vi "Get Bounds.vi"(8 "error in (no error)":errorcluster, 11 "Shape in":refnum<class "Shape.lvclass">) -> (0 "error out":errorcluster, 2 "Bounds":T1, 3 "Shape out":refnum<class "Shape.lvclass">)   [LabVIEW 2017, in "LV Image Editor Framework.lvlib" / "Shape.lvclass"]
uses:
  <vilib>/LIEF/Forms/Shape/Shape.lvclass
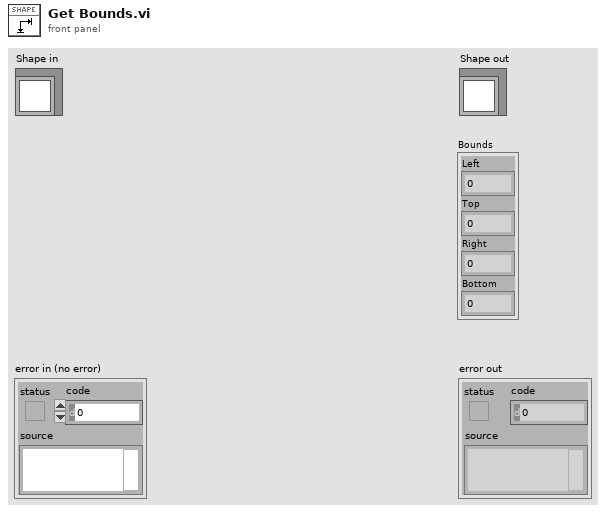
[diagram p1: front panel]
types:
  T1 = cluster{"Left":i32, "Top":i32, "Right":i32, "Bottom":i32}
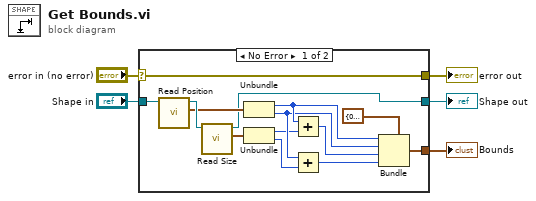
[diagram p0: block diagram]
diagram:
  n1 = case shown="No Error" "error in (no error)" {
    selector: "error in (no error)" -> [w19 w21]
    tunnel: [w19 w21] -> w4
    tunnel: [w6 w20] -> w2
    tunnel: "Shape in" -> [w13 w20]
    tunnel: [w15 _] -> w1
    frame No Error {
      n2 = call-dynamic "Read Position.vi"("Shape in"=w13) -> ("Position"=w12:cluster{"Left":i32, "Top":i32}, "Shape out"=w14:refnum<class "Shape.lvclass">)  [unwired: 8 in, 1 out]
      n3 = call-dynamic "Read Size.vi"("Shape in"=w14) -> ("Size"=w11:cluster{"Width":i32, "Height":i32}, "Shape out"=w6:refnum<class "Shape.lvclass">)  [unwired: 8 in, 1 out]
      n4 = Unbundle(w12) -> ("Left"=w10:i32, "Top"=w9:i32)
      n5 = Unbundle(w11) -> ("Width"=w8:i32, "Height"=w7:i32)
      n6 = Add(x=w10, y=w8) -> (x+y=w18:i32)
      n7 = Add(x=w9, y=w7) -> (x+y=w17:i32)
      n8 = Bundle(cluster=T1 {"Left"=0, "Top"=0, "Right"=0, "Bottom"=0} ("output cluster"), "Left"=w10, "Top"=w9, "Right"=w18, "Bottom"=w17) -> (w15:T1)
    }
    frame Error {
    }
  }
  "error out" <- w4
  "Shape out" <- w2
  "Bounds" <- w1
